vi "写入LoggerName.vi"(8 "error in (no error)":errorcluster caption="错误输入（无错误）", 10 "LoggerName":string, 11 "Logger输入":refnum<class "Logger.lvclass">) -> (0 "error out":errorcluster caption="错误输出", 3 "Logger输出":refnum<class "Logger.lvclass">)   [LabVIEW 2019, in "Logger.lvclass"]
uses:
  <userlib>/Logger/Logger.lvclass
  <userlib>/Logger/Logger.lvclass/Logger.ctl
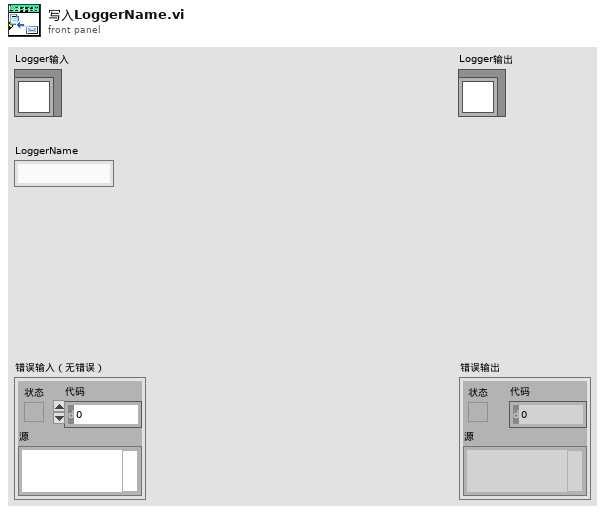
[diagram p1: front panel]
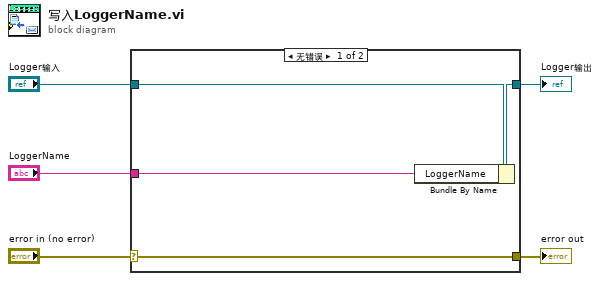
[diagram p0: block diagram]
diagram:
  n1 = case shown="无错误" "error in (no error)" {
    selector: "error in (no error)" -> [w9 w10]
    tunnel: [w9 w10] -> w4
    tunnel: [w7 w11] -> w2
    tunnel: "Logger输入" -> [w8 w11]
    tunnel: "LoggerName" -> [w6 _]
    frame No Error {
      n2 = Bundle By Name(cluster=w8, "LoggerName"=w6) -> (w7:refnum<class "Logger.lvclass">)
    }
    frame Error {
    }
  }
  "error out" <- w4
  "Logger输出" <- w2
